vi "Teleop.vi"(10 "Match Info":T1={"Autonomous Elapsed Seconds"=0.0, "TeleOp Elapsed Seconds"=0.0, "Disabled Elapsed Seconds"=0.0, "Visited Autonomous"=FALSE, "Visited TeleOp"=FALSE, "Visited Disabled"=FALSE, "Autonomous Settings"={"Autonomous Style"=enum."Independent", "VI Refnum"=refnum}}, 11 "Call Context":T2) -> ()   [LabVIEW 2016]
doc: "This VI is called for each TeleOp packet received from the DS where the robot is not disabled. It is often used to read from the joysticks and update I/O or to update setpoints for timed control loops. It should complete and return within 20 milliseconds or it may miss DS packets."
uses:
  <vilib>/Rock Robotics/WPI/DriverStation/WPI_DriverStationDerivedRobotMode.ctl
  <vilib>/Rock Robotics/WPI/DriverStation/WPI_DriverStationMatch Info.ctl
  Sprocket/src/Refname/Joysticks.ctl
  Sprocket/src/Action/Action Name.ctl
  Sprocket/src/Refname/Queues.ctl
  Sprocket/src/Refname/Refname to String (Queue).vi
  Sprocket/src/Refname/Refname to String (Joystick).vi
  Robot Global Data.vi
  <vilib>/Rock Robotics/WPI/Utilities/WPI_GetSetVariantRefNum.vi
  Sprocket/src/Stream/Push Stream.vi
  Sprocket/src/Stream/Release Stream.vi
  Sprocket/lib/Sprocket.lvlib
panel:
  in  "Right Side Scale":dbl=0.93
  in  "LowGearMotorScale":dbl=0.7 format="%#_13g"
  in  "Wedge speed divider":dbl=1.5
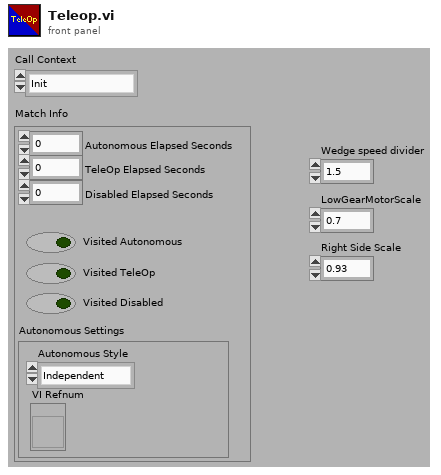
[diagram p1: front panel]
types:
  T1 = typedef "WPI_DriverStationMatch Info.ctl" = cluster{"Autonomous Elapsed Seconds":dbl, "TeleOp Elapsed Seconds":dbl, "Disabled Elapsed Seconds":dbl, "Visited Autonomous":bool, "Visited TeleOp":bool, "Visited Disabled":bool, "Autonomous Settings":cluster{"Autonomous Style":enum16{"Iterative", "Independent"}, "VI Refnum":refnum<vi>}}
  T2 = typedef "WPI_DriverStationDerivedRobotMode.ctl" = enum16{"Init", "Execute", "Stop"}
  T3 = typedef "Sprocket.lvlib/Action Name.ctl" = enum16{"No Action", "Drive Train Both", "Drive Train Rotate", "Drive Train Throttle", "Collector Motor Roll", "Collector Motor Eject", "Collector Motor Collect", "Collector Motor Stop", "Collector Extend", "Collector Retract", "Shifter High", "Shifter Low", "Collector Motor Stall", "Wedge Roll"}
  T4 = typedef "Sprocket.lvlib/Joysticks.ctl" = enum16{"Joystick 0", "Joystick 1", "Joystick 2", "Joystick 3"}
  T5 = typedef "Sprocket.lvlib/Queues.ctl" = enum16{"Input", "Drive", "Collector", "Shifter", "Wedge"}
  T6 = typedef "WPI_JoystickDevRef.ctl" = cluster{"Device":T7}
  T7 = typedef "WPI_JoystickDeviceEnum.ctl" = enum16{"USB 0", "USB 1", "USB 2", "USB 3", "USB 4", "USB 5"}
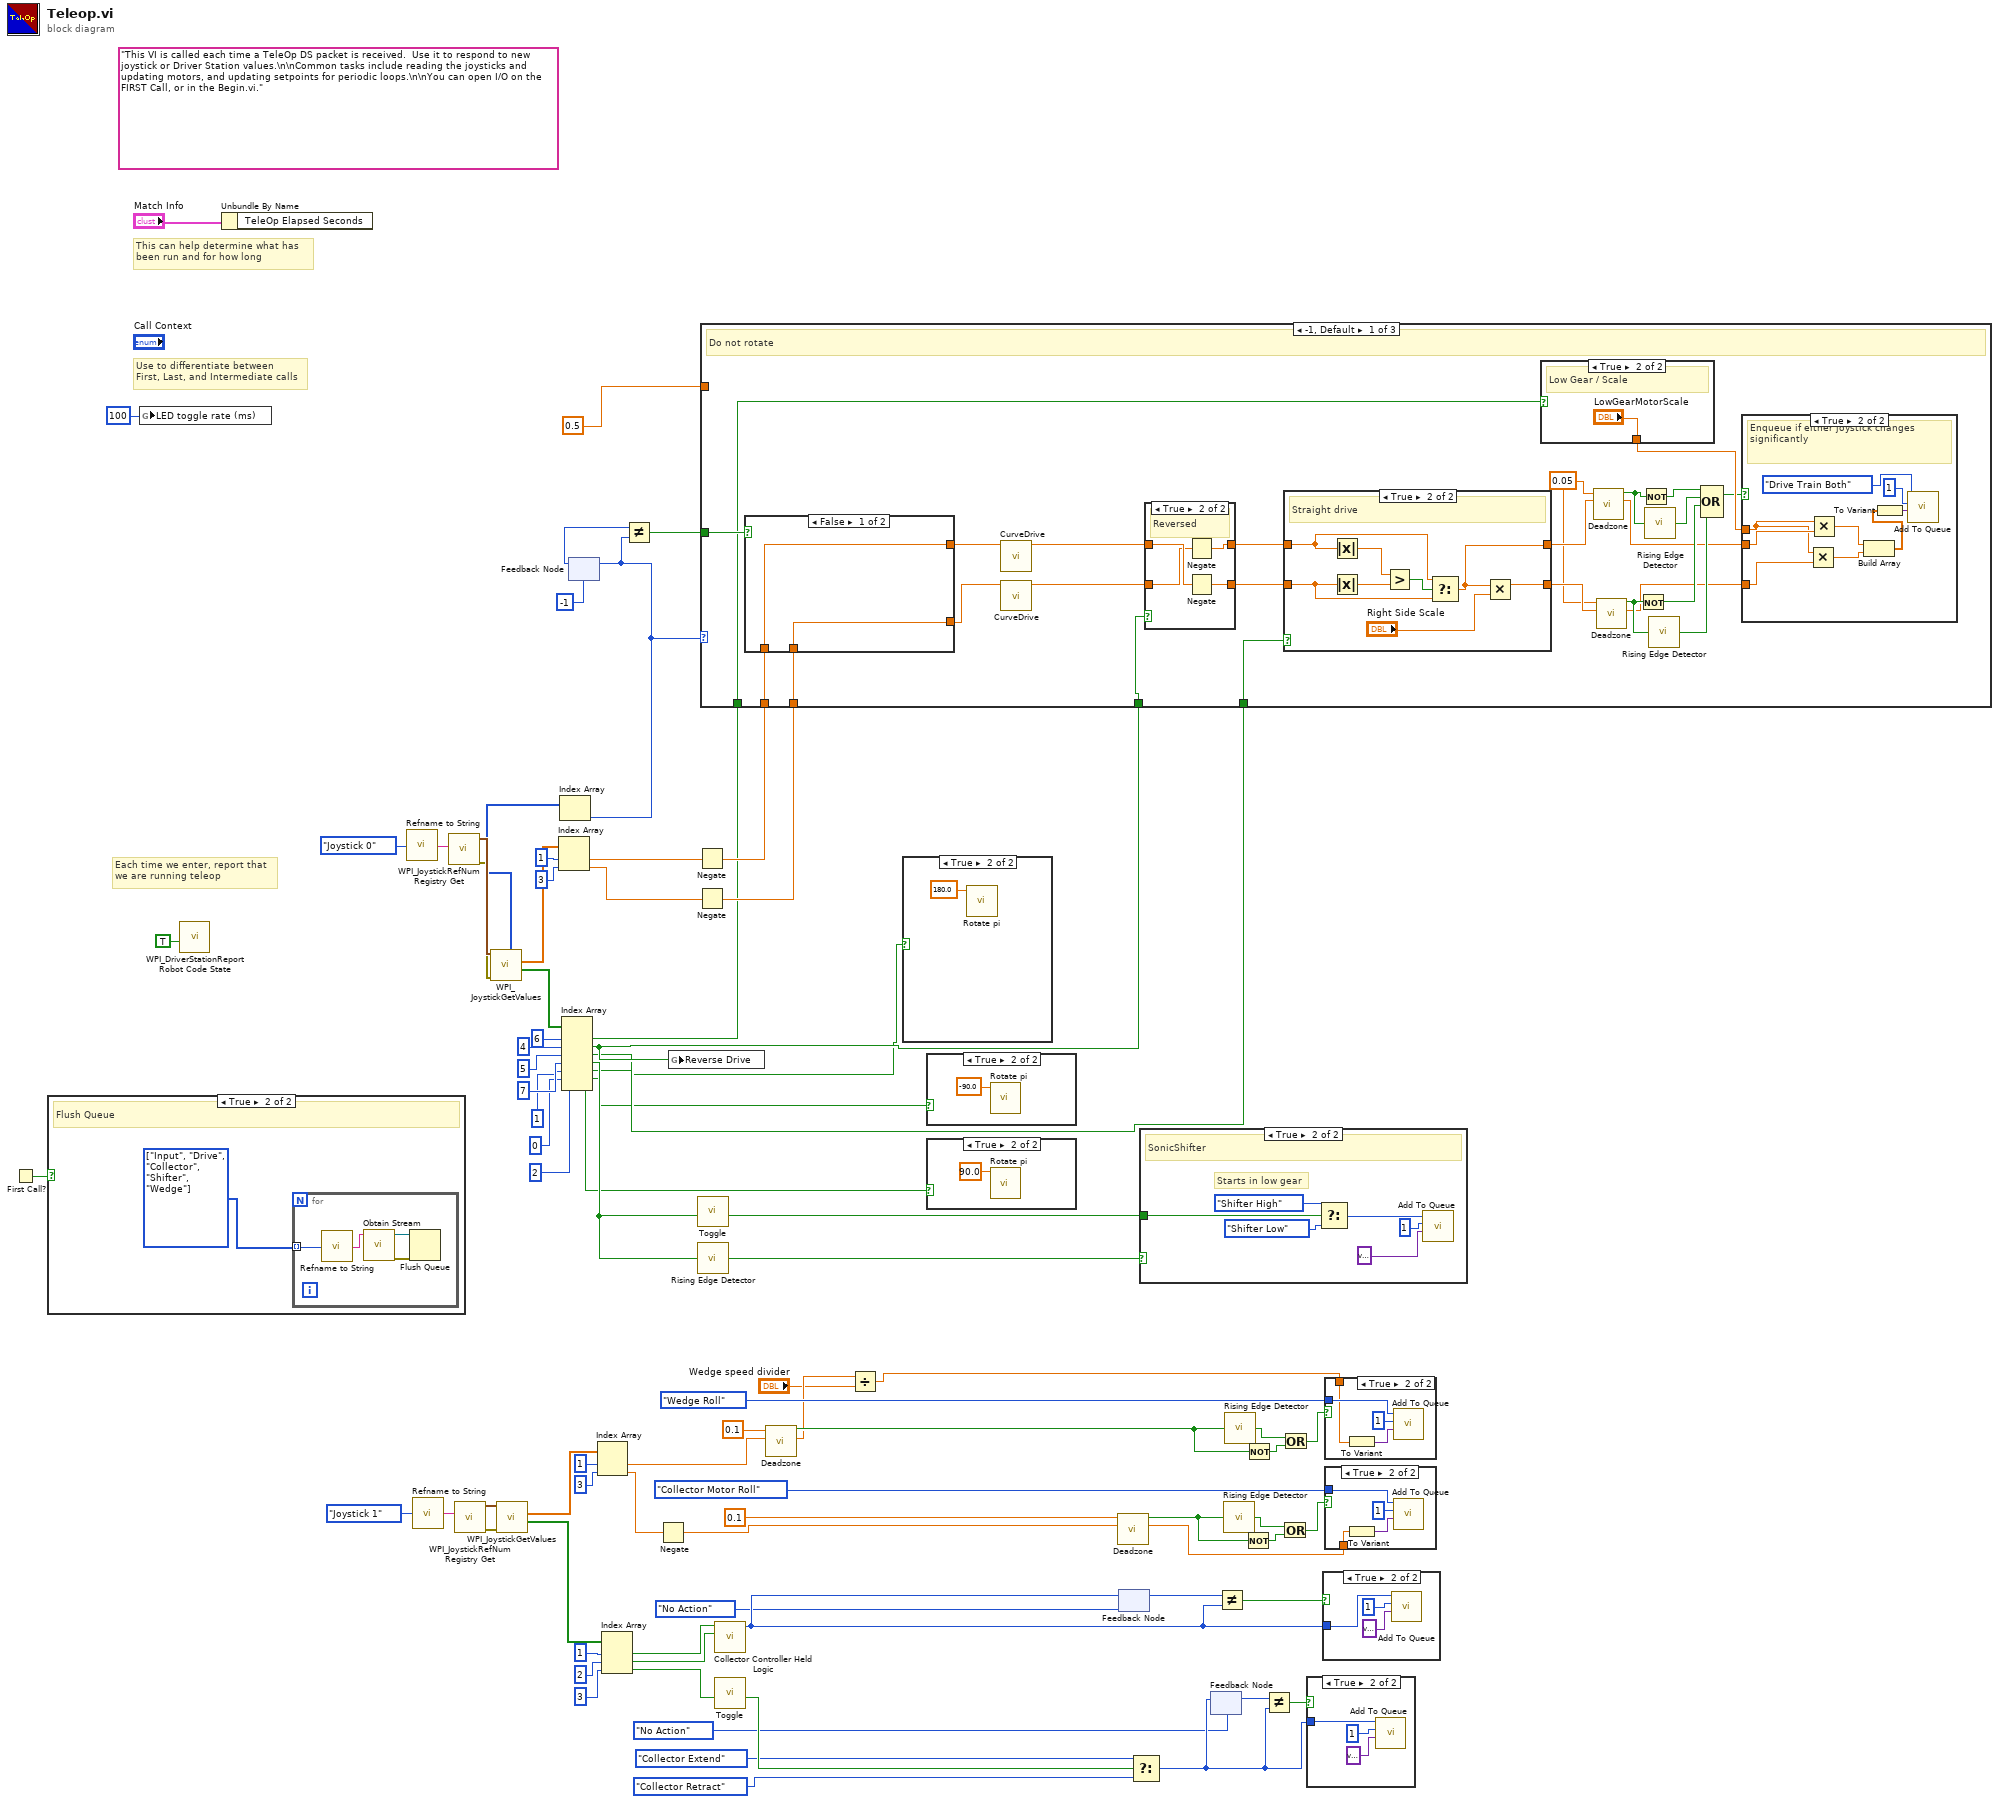
[diagram p0: block diagram]
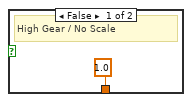
[diagram p5: hidden frame]
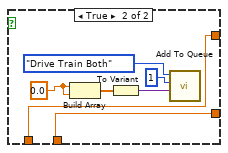
[diagram p6: hidden frame]
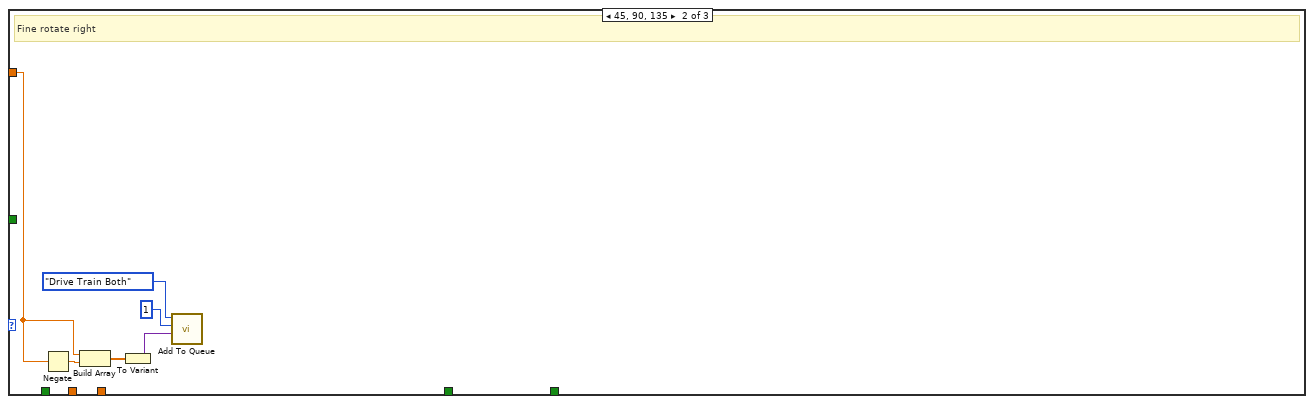
[diagram p10: hidden frame]
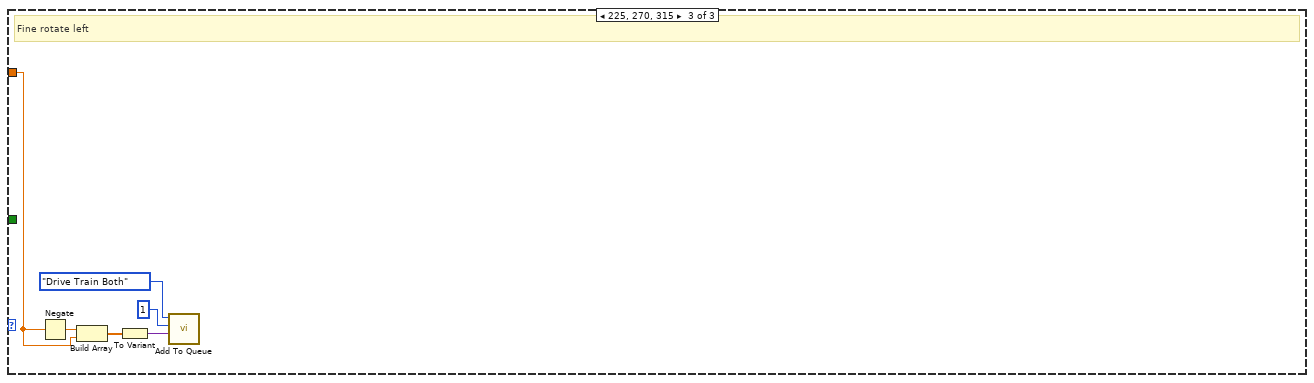
[diagram p11: hidden frame]
diagram:
  (unwired) "This VI is called each time a TeleOp DS packet is received.  Use it to respond to new joystick or Driver Station values.\n\nCommon tasks include reading the joysticks and updating motors, and updating setpoints for periodic loops.\n\nYou can open I/O on the FIRST Call, or in the Begin.vi."
  # "Each time we enter, report that\nwe are running teleop"
  # "Use to differentiate between\nFirst, Last, and Intermediate calls"
  # "This can help determine what has\nbeen run and for how long"
  n1 = First Call?() -> (First Call?: T/F=w47:bool)
  n2 = case shown="True" w47 {
    frame False {
    }
    frame True {
      w83 = T5[] [enum."Input", enum."Drive", enum."Collector", enum."Shifter", enum."Wedge"] items=["Input", "Drive", "Collector", "Shifter", "Wedge"]
      # "Flush Queue"
      n3 = for {
        tunnel: w83 -> [w84] mode=indexing
        n4 = call-poly "Refname to String.vi"("Queue Refname"=w84) -> ("Refnum Name"=w85:string)
        n5 = call "Obtain Stream.vi"("Name"=w85) -> ("error out"=w87:errorcluster, "stream out"=w86:refnum<queue>)  [unwired: 9 in]
        n6 = Flush Queue(queue=w86, error in (no error)=w87) -> ()  [unwired: 3 out]
      }
    }
  }
  n7 = global write "Robot Global Data.vi" "LED toggle rate (ms)"(u32 100 ("LED toggle rate (ms)")) -> ()
  n8 = call <vilib>:"WPI_DriverStationReport Robot Code State.vi"("TeleOp"=TRUE ("Autonomous")) -> ()  [unwired: 10 in, 1 out]
  n9 = Unbundle By Name("Match Info") -> ()  [unwired: 1 out]
  n10 = call-poly "Refname to String.vi"("Joystick Refname"=Joysticks."Joystick 0") -> ("Refnum Name"=w76:string)
  n11 = call-poly "Refname to String.vi"("Joystick Refname"=Joysticks."Joystick 1") -> ("Refnum Name"=w67:string)
  n12 = call <vilib>:"WPI_JoystickRefNum Registry Get.vi"("refnum name"=w76) -> ("error out"=w78:errorcluster, "JoystickDevRef"=w79:T6)  [unwired: 9 in]
  n13 = call <vilib>:"WPI_JoystickRefNum Registry Get.vi"("refnum name"=w67) -> ("error out"=w65:errorcluster, "JoystickDevRef"=w64:T6)  [unwired: 9 in]
  n14 = call <vilib>:"WPI_JoystickGetValues.vi"("error in (no error)"=w78, "JoystickDevRef"=w79) -> ("Buttons"=w8:bool[], "Axes"=w75:dbl[], "POVs"=w32:i16[])  [unwired: 5 in, 2 out]
  n15 = call <vilib>:"WPI_JoystickGetValues.vi"("error in (no error)"=w65, "JoystickDevRef"=w64) -> ("Buttons"=w63:bool[], "Axes"=w68:dbl[])  [unwired: 5 in, 3 out]
  n16 = Index Array(array=w75, index #1=1 ("index"), index #2=3 ("index")) -> (element #1=w71:dbl, element #2=w72:dbl)
  n17 = Index Array(array=w32) -> (element=w26:i16)  [unwired: 1 in]
  n18 = Index Array(array=w8, index #1=6 ("index"), index #2=4 ("index"), index #3=5 ("index"), index #4=7 ("index"), index #5=1 ("index"), index #6=0 ("index"), index #7=2 ("index")) -> (element #1=w15:bool, element #2=w14:bool, element #3=w13:bool, element #4=w12:bool, element #5=w11:bool, element #6=w10:bool, element #7=w9:bool)
  n19 = feedback-in #1(w26) -> ()
  n20 = feedback #1(-1) -> (w28:i32)
  n21 = Index Array(array=w68, index #1=1 ("index"), index #2=3 ("index")) -> (element #1=w38:dbl, element #2=w42:dbl)
  n22 = Index Array(array=w63, index #1=1 ("index"), index #2=2 ("index"), index #3=3 ("index")) -> (element #1=w60:bool, element #2=w59:bool, element #3=w56:bool)
  n23 = Not Equal?(x=w28, y=w26) -> (x != y?=w25:bool)
  n24 = Negate(x=w42) -> (-x=w33:dbl)
  n25 = global write "Robot Global Data.vi" "Reverse Drive"(w14) -> ()
  n26 = Negate(x=w71) -> (-x=w30:dbl)
  n27 = Negate(x=w72) -> (-x=w29:dbl)
  n28 = call "Toggle.vi"("Input"=w12) -> ("Toggled output"=w55:bool)  [unwired: 10 in]
  n29 = call "Rising Edge Detector.vi"("Input"=w12) -> ("Rising edge?"=w54:bool)
  n30 = case shown="-1, Default" w26 {
    tunnel: 0.5 -> [_ w150 w156]
    tunnel: w14 -> [w89 _ _]
    tunnel: w13 -> [w108 _ _]
    tunnel: w30 -> [w106 _ _]
    tunnel: w29 -> [w105 _ _]
    tunnel: w25 -> [w107 _ _]
    tunnel: w15 -> [w88 _ _]
    frame -1, Default {
      w99 = 0.05 ("Deadzone")
      # "Do not rotate"
      n31 = case shown="False" w107 {
        tunnel: w106 -> [w116 w119]
        tunnel: w105 -> [w115 w118]
        tunnel: [w116 w119] -> w104
        tunnel: [w115 w118] -> w103
        frame False {
        }
        frame True {
          w120 = 0.0
          n32 = Build Array(w120, w120) -> (w123:dbl[])
          n33 = To Variant(anything=w123) -> (Variant=w122:variant)
          n34 = call "Add To Queue.vi"("Data"=w122, "Priority"=1, "Action"=Action_Name."Drive Train Both" ("Name")) -> ()  [unwired: 8 in, 1 out]
        }
      }
      n35 = call "CurveDrive.vi"("Joystick"=w104) -> ("Throttle"=w112:dbl)  [unwired: 9 in, 1 out]
      n36 = call "CurveDrive.vi"("Joystick"=w103) -> ("Throttle"=w111:dbl)  [unwired: 9 in, 1 out]
      n37 = case shown="True" w89 {
        tunnel: w112 -> [w133 w138]
        tunnel: w111 -> [w134 w137]
        tunnel: [w133 w136] -> w110
        tunnel: [w134 w135] -> w109
        frame False {
          # "Normal"
        }
        frame True {
          # "Reversed"
          n38 = Negate(x=w137) -> (-x=w136:dbl)
          n39 = Negate(x=w138) -> (-x=w135:dbl)
        }
      }
      n40 = case shown="True" w108 {
        tunnel: [w139 w147] -> w101
        tunnel: w110 -> [w139 w144]
        tunnel: w109 -> [w140 w148]
        tunnel: [w140 w142] -> w100
        frame False {
          # "Normal"
        }
        frame True {
          # "Straight drive"
          n41 = Absolute Value(x=w144) -> (abs(x)=w145:dbl)
          n42 = Absolute Value(x=w148) -> (abs(x)=w143:dbl)
          n43 = Greater?(x=w145, y=w143) -> (0:w146:bool)
          n44 = Select(t=w144, s=w146, f=w148) -> (s? t:f=w147:dbl)
          n45 = Multiply(x=w147, y="Right Side Scale") -> (x*y=w142:dbl)
        }
      }
      n46 = case shown="True" w88 {
        tunnel: [1.0 ("LowGearMotorScale") "LowGearMotorScale"] -> w102
        frame False {
          # "High Gear / No Scale"
        }
        frame True {
          # "Low Gear / Scale"
        }
      }
      n47 = call "Deadzone.vi"("Input"=w101, "Deadzone"=w99) -> ("Output"=w91:dbl, "In deadzone?"=w98:bool)  [unwired: 7 in, 1 out]
      n48 = call "Deadzone.vi"("Input"=w100, "Deadzone"=w99) -> ("Output"=w90:dbl, "In deadzone?"=w97:bool)  [unwired: 7 in, 1 out]
      n49 = Not(x=w97) -> (.not. x?=w94:bool)
      n50 = Not(x=w98) -> (.not. x?=w96:bool)
      n51 = call "Rising Edge Detector.vi"("Input"=w98) -> ("Rising edge?"=w95:bool)
      n52 = call "Rising Edge Detector.vi"("Input"=w97) -> ("Rising edge?"=w93:bool)
      n53 = Compound Arithmetic op=OR(w96, w95, w94, w93) -> (w92:bool)
      n54 = case shown="True" w92 {
        tunnel: w91 -> [_ w129]
        tunnel: w90 -> [_ w125]
        tunnel: w102 -> [_ w127]
        frame False {
        }
        frame True {
          # "Enqueue if either joystick changes significantly"
          n55 = Multiply(x=w127, y=w125) -> (x*y=w126:dbl)
          n56 = Multiply(x=w127, y=w129) -> (x*y=w128:dbl)
          n57 = Build Array(w128, w126) -> (w132:dbl[])
          n58 = To Variant(anything=w132) -> (Variant=w131:variant)
          n59 = call "Add To Queue.vi"("Data"=w131, "Priority"=1, "Action"=Action_Name."Drive Train Both" ("Name")) -> ()  [unwired: 8 in, 1 out]
        }
      }
    }
    frame 45, 90, 135 {
      # "Fine rotate right"
      n60 = Negate(x=w150) -> (-x=w151:dbl)
      n61 = Build Array(w150, w151) -> (w154:dbl[])
      n62 = To Variant(anything=w154) -> (Variant=w153:variant)
      n63 = call "Add To Queue.vi"("Data"=w153, "Priority"=1, "Action"=Action_Name."Drive Train Both" ("Name")) -> ()  [unwired: 8 in, 1 out]
    }
    frame 225, 270, 315 {
      # "Fine rotate left"
      n64 = Negate(x=w156) -> (-x=w157:dbl)
      n65 = Build Array(w157, w156) -> (w160:dbl[])
      n66 = To Variant(anything=w160) -> (Variant=w159:variant)
      n67 = call "Add To Queue.vi"("Data"=w159, "Priority"=1, "Action"=Action_Name."Drive Train Both" ("Name")) -> ()  [unwired: 8 in, 1 out]
    }
  }
  n68 = call "Collector Controller Held Logic.vi"("Button B"=w59, "Button A"=w60) -> ("State out"=w51:T3)  [unwired: 9 in]
  n69 = call "Toggle.vi"("Input"=w56) -> ("Toggled output"=w57:bool)  [unwired: 10 in]
  n70 = call "Deadzone.vi"("Input"=w38, "Deadzone"=0.1) -> ("Output"=w17:dbl, "In deadzone?"=w35:bool)  [unwired: 7 in, 1 out]
  n71 = Divide(x=w17, y="Wedge speed divider") -> (x/y=w18:dbl)
  n72 = case shown="True" w11 {
    frame False {
    }
    frame True {
      n73 = call "Rotate pi.vi"("Degrees"=180.0) -> ()  [unwired: 11 in]
    }
  }
  n74 = case shown="True" w10 {
    frame False {
    }
    frame True {
      n75 = call "Rotate pi.vi"("Degrees"=-90.0) -> ()  [unwired: 11 in]
    }
  }
  n76 = case shown="True" w9 {
    frame False {
    }
    frame True {
      n77 = call "Rotate pi.vi"("Degrees"=90.0) -> ()  [unwired: 11 in]
    }
  }
  n78 = call "Deadzone.vi"("Input"=w33, "Deadzone"=0.1) -> ("Output"=w41:dbl, "In deadzone?"=w44:bool)  [unwired: 7 in, 1 out]
  n79 = feedback-in #2(w51) -> ()
  n80 = feedback #2(Action_Name."No Action" ("Name")) -> (w53:T3)
  n81 = Select(t=Action_Name."Collector Extend" ("Name"), s=w57, f=Action_Name."Collector Retract" ("Name")) -> (s? t:f=w48:T3)
  n82 = case shown="True" w54 {
    tunnel: w55 -> [_ w169]
    frame False {
    }
    frame True {
      # "Starts in low gear"
      # "SonicShifter"
      n83 = Select(t=Action_Name."Shifter High" ("Name"), s=w169, f=Action_Name."Shifter Low" ("Name")) -> (s? t:f=w167:T3)
      n84 = call "Add To Queue.vi"("Data"=variant, "Priority"=1, "Action"=w167) -> ()  [unwired: 8 in, 1 out]
    }
  }
  n85 = feedback-in #3(w48) -> ()
  n86 = feedback #3(Action_Name."No Action" ("Name")) -> (w50:T3)
  n87 = Not Equal?(x=w53, y=w51) -> (x != y?=w52:bool)
  n88 = call "Rising Edge Detector.vi"("Input"=w44) -> ("Rising edge?"=w43:bool)
  n89 = call "Rising Edge Detector.vi"("Input"=w35) -> ("Rising edge?"=w37:bool)
  n90 = Not(x=w44) -> (.not. x?=w45:bool)
  n91 = Not(x=w35) -> (.not. x?=w36:bool)
  n92 = Not Equal?(x=w50, y=w48) -> (x != y?=w49:bool)
  n93 = Or(x=w43, y=w45) -> (x .or. y?=w40:bool)
  n94 = Or(x=w37, y=w36) -> (x .or. y?=w34:bool)
  n95 = case shown="True" w49 {
    tunnel: w48 -> [_ w170]
    frame False {
    }
    frame True {
      n96 = call "Add To Queue.vi"("Data"=variant, "Priority"=1, "Action"=w170) -> ()  [unwired: 8 in, 1 out]
    }
  }
  n97 = case shown="True" w52 {
    tunnel: w51 -> [_ w173]
    frame False {
    }
    frame True {
      n98 = call "Add To Queue.vi"("Data"=variant, "Priority"=1, "Action"=w173) -> ()  [unwired: 8 in, 1 out]
    }
  }
  n99 = case shown="True" w34 {
    tunnel: Action_Name."Wedge Roll" ("Name") -> [_ w179]
    tunnel: w18 -> [_ w177]
    frame False {
    }
    frame True {
      n100 = To Variant(anything=w177) -> (Variant=w176:variant)
      n101 = call "Add To Queue.vi"("Data"=w176, "Priority"=1, "Action"=w179) -> ()  [unwired: 8 in, 1 out]
    }
  }
  n102 = case shown="True" w40 {
    tunnel: Action_Name."Collector Motor Roll" ("Name") -> [_ w183]
    tunnel: w41 -> [_ w181]
    frame False {
    }
    frame True {
      n103 = To Variant(anything=w181) -> (Variant=w180:variant)
      n104 = call "Add To Queue.vi"("Data"=w180, "Priority"=1, "Action"=w183) -> ()  [unwired: 8 in, 1 out]
    }
  }
